vi "Get Bucket Location.vi"(8 "error in (no error)":errorcluster, 11 "Bucket in":refnum<class "Bucket.lvclass">) -> (0 "error out":errorcluster, 2 "Location":T1, 3 "Bucket out":refnum<class "Bucket.lvclass">)   [LabVIEW 2015, in "NI_AWS_S3.lvlib" / "Bucket.lvclass"]
uses:
  Bucket.lvclass
  Core/HTTP Request/Region.ctl
  Core/HTTP Request/Request Options.ctl
  Core/HTTP Request/Name Value Pair.ctl
  Core/HTTP Request/Region handling.ctl
  Core/HTTP Request/URL formatting.ctl
  Bucket.lvclass/Bucket.ctl
  Read Name.vi
  Core/HTTP Request/HTTP Request.lvclass
  NI_AWS_S3.lvlib
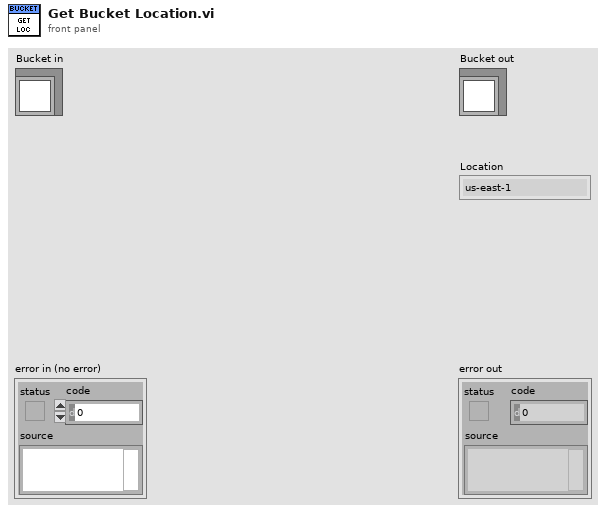
[diagram p1: front panel]
types:
  T1 = typedef "NI_AWS_Core.lvlib/HTTP Request.lvclass/Region.ctl" = enum16{"us-east-1", "us-east-2", "us-west-1", "us-west-2", "ap-northeast-1", "ap-northeast-2", "ap-southeast-1", "ap-southeast-2", "ca-central-1", "eu-central-1", "eu-west-1", "eu-west-2", "sa-east-1"}
  T2 = typedef "NI_AWS_S3.lvlib/URL formatting.ctl" = enum16{"region-", "region."}
  T3 = typedef "NI_AWS_S3.lvlib/Region handling.ctl" = enum16{"use region everywhere", "use region (authentication only)", "use region (URL only)", "ignore region everwhere"}
  T4 = typedef "NI_AWS_Core.lvlib/HTTP Request.lvclass/Name Value Pair.ctl" = cluster{"name":string, "value":string}
  T5 = typedef "NI_AWS_Core.lvlib/HTTP Request.lvclass/Request Options.ctl" = cluster{"request headers":T4[], "request parameters":T4[], "request body":string, "region handling":T3, "URL formatting":T2}
  T6 = typedef "NI_AWS_Core.lvlib/HTTP Request.lvclass/Response.ctl" = cluster{"Headers":string, "Body":string}
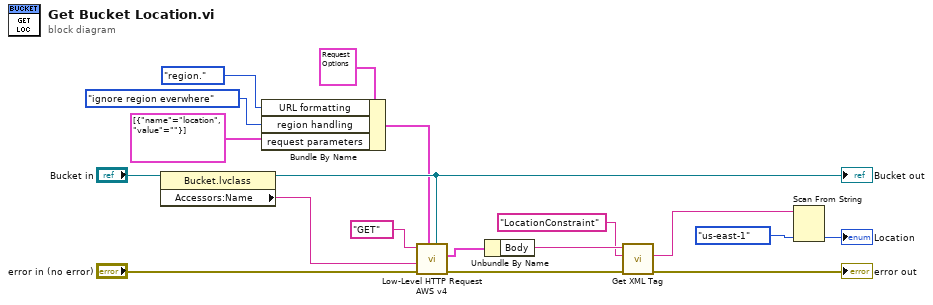
[diagram p0: block diagram]
diagram:
  n1 = property class="Bucket.lvclass"(reference="Bucket in") -> (reference out=w15:refnum<class "Bucket.lvclass">, "Accessors:Name"=w3:string)  [unwired: 1 in, 1 out]
  "Bucket out" <- w15
  n2 = Bundle By Name(cluster=T5 {"request headers"=[], "request parameters"=[], "request body"="", "region handling"=enum."use region everywhere", "URL formatting"=enum."region."} ("Request Options"), "URL formatting"=URL_formatting."region.", "region handling"=Region_handling."ignore region everwhere", "request parameters"=T4[] [{"name"="location", "value"=""}]) -> (w4:T5)
  n3 = call "Low-Level HTTP Request AWS v4.vi"("AWS Core"=w15, "Request Options"=w4, "error in (no error)"="error in (no error)", "URL Suffix"=w3, "HTTP-Verb"="GET") -> ("error out"=w11:errorcluster, "Response"=w13:T6)  [unwired: 4 in, 1 out]
  n4 = Unbundle By Name(w13) -> ("Body"=w12:string)
  n5 = call "Get XML Tag.vi"("error in (no error)"=w11, "Tag name"="LocationConstraint", "XML String in"=w12) -> ("error out"=→"error out":errorcluster, "Tag value"=w8:string)  [unwired: 4 in, 3 out]
  n6 = Scan From String(input string=w8, default 1=Region."us-east-1" ("Region")) -> (output 1=→"Location":T1)  [unwired: 3 in, 3 out]
